vi "Initialize.vi"(7 "image path":path=path "<Not a Path>", 8 "error in":errorcluster, 10 "DataGridView":refnum<k24>(container), 11 "DataGrid in":refnum<class "DataGridView.lvclass">) -> (0 "error out":errorcluster, 3 "DataGrid out":refnum<class "DataGridView.lvclass">)   [LabVIEW 2016, in "DataGrid.lvlib" / "DataGridView.lvclass"]
doc: "Sets all the initial default values of various properties to make a datagrid more user friendly. These can be modified thorugh the class properties, they are simple all set together in this default initialization.\n\nOptionally, add the image path to specify any folder of images to use. If that is not specified, the application folder / images is used to search for image file references."
uses:
  <userlib>/LabVIEWdotNetDataGrid/source/DataGridView/DataGridView.lvclass
  System.Windows.Forms
  <userlib>/LabVIEWdotNetDataGrid/source/DataGridView/DataGridView.lvclass/DataGridView.ctl
  <userlib>/LabVIEWdotNetDataGrid/source/DataGridView/Properties/Write AllowUserToResizeRows.vi
  <userlib>/LabVIEWdotNetDataGrid/source/DataGridView/Properties/Write AllowUserToAddRows.vi
  <userlib>/LabVIEWdotNetDataGrid/source/DataGridView/Properties/Write AllowUserToDeleteRows.vi
  <userlib>/LabVIEWdotNetDataGrid/source/DataGridView/Properties/Write AllowUserToResizeColumns.vi
  <userlib>/LabVIEWdotNetDataGrid/source/DataGridView/Properties/Write RowHeadersVisible.vi
  <userlib>/LabVIEWdotNetDataGrid/source/DataGridView/Properties/Write AutoSizeColumnsMode.vi
  <userlib>/LabVIEWdotNetDataGrid/source/DataGridView/Properties/Write AutoSizeRowsMode.vi
  <userlib>/LabVIEWdotNetDataGrid/source/DataGridView/Properties/Write DefaultCellBGKColor.vi
  <userlib>/LabVIEWdotNetDataGrid/source/DataGridView/Properties/Write DefaultAlternateCellBGKColor.vi
  <userlib>/LabVIEWdotNetDataGrid/source/DataGridView/Properties/Write SelectionMode.vi
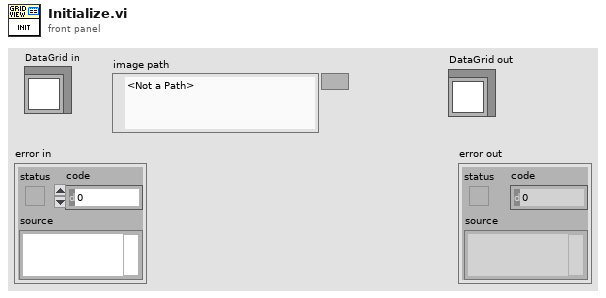
[diagram p1: front panel]
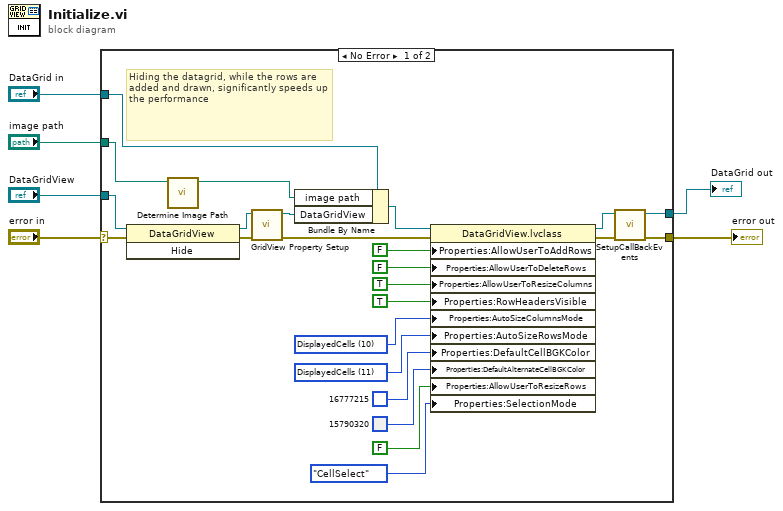
[diagram p0: block diagram]
diagram:
  n1 = case shown="No Error" "error in" {
    selector: "error in" -> [w27 w32]
    tunnel: [w29 w32] -> w5
    tunnel: [w28 w31] -> w3
    tunnel: "DataGrid in" -> [w30 w31]
    tunnel: "DataGridView" -> [w26 _]
    tunnel: "image path" -> [w10 _]
    frame No Error {
      w18 = 11 items=["None"=0, "AllHeaders"=5, "AllCellsExceptHeaders"=6, "AllCells"=7, "DisplayedHeaders"=9, "DisplayedCellsExceptHeaders"=10, "DisplayedCells"=11] ("AutoSizeRowsMode")
      w19 = 10 items=["None"=1, "ColumnHeader"=2, "AllCellsExceptHeader"=4, "AllCells"=6, "DisplayedCellsExceptHeader"=8, "DisplayedCells"=10, "Fill"=16] ("AutoSizeColumnsMode")
      # "Hiding the datagrid, while the rows are added and drawn, significantly speeds up the performance"
      n2 = invoke class="DataGridView" method="Hide"(reference=w26, error in=w27) -> (reference out=w23:refnum<k24>, error out=w25:errorcluster)  [unwired: 1 in, 1 out]
      n3 = call <userlib>:"Determine Image Path.vi"("image path"=w10) -> ("Path"=w9:path)  [unwired: 10 in]
      n4 = call <userlib>:"GridView Property Setup.vi"("error in (no error)"=w25, ".NET Refnum in"=w23) -> ("error out"=w24:errorcluster, ".NET Refnum out"=w22:refnum<k24>)  [unwired: 8 in]
      n5 = Bundle By Name(cluster=w30, "image path"=w9, "DataGridView"=w22) -> (w20:refnum<class "DataGridView.lvclass">)
      n6 = property class="DataGridView.lvclass"(reference=w20, error in=w24, "Properties:AllowUserToAddRows"=FALSE ("AllowUserToAddRows"), "Properties:AllowUserToDeleteRows"=FALSE ("AllowUserToDeleteRows"), "Properties:AllowUserToResizeColumns"=TRUE ("AllowUserToResizeColumns"), "Properties:RowHeadersVisible"=TRUE ("RowHeadersVisible"), "Properties:AutoSizeColumnsMode"=w19, "Properties:AutoSizeRowsMode"=w18, "Properties:DefaultCellBGKColor"=u32 16777215, "Properties:DefaultAlternateCellBGKColor"=u32 15790320, "Properties:AllowUserToResizeRows"=FALSE ("AllowUserToResizeRows"), "Properties:SelectionMode"=enum16{"CellSelect", "FullRowSelect"}."CellSelect" ("SelectionMode")) -> (reference out=w15:refnum<class "DataGridView.lvclass">, error out=w14:errorcluster)
      n7 = call <userlib>:"SetupCallBackEvents.vi"("error in (no error)"=w14, "DataGridView in"=w15) -> ("error out"=w29:errorcluster, "DataGridView out"=w28:refnum<class "DataGridView.lvclass">)  [unwired: 8 in]
    }
    frame Error {
    }
  }
  "error out" <- w5
  "DataGrid out" <- w3
